vi "NET SetHalideScheduler.vi"(8 "error in (no error)":errorcluster, 10 "Scheduler":path, 11 "NET in":refnum<class "NET.lvclass">) -> (0 "error out":errorcluster, 3 "NET out":refnum<class "NET.lvclass">)   [LabVIEW 2020, in "OpenLvVision_OpenCv.lvlib" / "NET.lvclass"]
doc: "Compile Halide layers. \nSchedule layers that support Halide backend. Then compile them for specific target. For layers that not represented in scheduling file or if no manual scheduling used at all, automatic scheduling will be applied."
uses:
  NET.lvclass
  C:/Users/lukas/Downloads/OpenLvVision_OpenCv/SourceCode/LabView/OpenLvVision_OpenCv/_LvHelpers/EdvrObject/EdvrObject.lvclass
  _LvHelpers/EdvrObject/EdvrObject.lvclass/EdvrObject.ctl
  OpenLvVision_OpenCv.lvlib
  _LvHelpers/EdvrObject/EdvrObject.lvclass
  Dlls/OlvOpenCvWrapper.dll
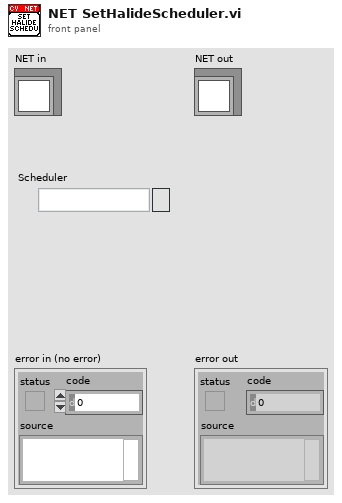
[diagram p1: front panel]
types:
  T1 = typedef "OpenLvVision_OpenCv.lvlib/EdvrObject.lvclass/Edvr.ctl" = refnum<data-value>
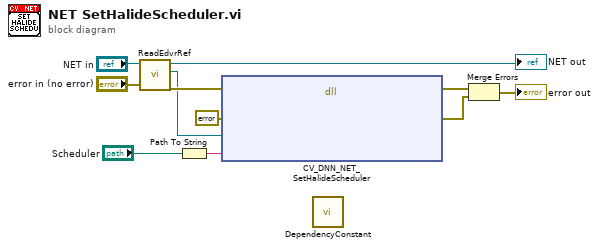
[diagram p0: block diagram]
diagram:
  n1 = call "ReadEdvrRef.vi"("error in (no error)"="error in (no error)", "EdvrObject in"="NET in") -> ("error out"=w7:errorcluster, "Edvr"=w6:T1, "EdvrObject out"=→"NET out":refnum<class "NET.lvclass">)  [unwired: 7 in]
  n2 = Path To String(path="Scheduler") -> (string=w2:string)
  n3 = dll-call lib="C:/Users/lukas/Downloads/OpenLvVision_OpenCv/SourceCode/LabView/OpenLvVision_OpenCv/Dlls/OlvOpenCvWrapper.dll" fn="CV_DNN_NET_SetHalideScheduler"(error in=w7, "Error"=errorcluster {"status"=FALSE, "code"=0, "source"=""} ("error out"), "edvrRef"=w6, "inputName"=w2) -> (error out=w10:errorcluster, "Error"=w3:errorcluster)  [unwired: 5 in, 1 out]
  n4 = call "DependencyConstant.vi"() -> ()  [unwired: 12 in]
  n5 = Merge Errors(w10, w3) -> (→"error out":errorcluster)
